vi "paramget.vi"(8 "dwLen":u32, 10 "byPara":u8) -> (1 "data out":u8[](array[numeric]), 2 "return":i32)   [LabVIEW 2016]
panel:
  in  "cmd_std_header_t":T1
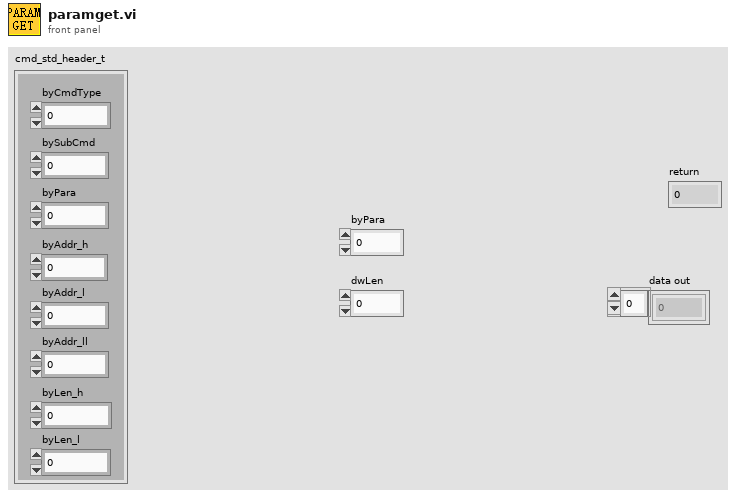
[diagram p1: front panel]
types:
  T1 = cluster{"byCmdType":u8, "bySubCmd":u8, "byPara":u8, "byAddr_h":u8, "byAddr_l":u8, "byAddr_ll":u8, "byLen_h":u8, "byLen_l":u8}
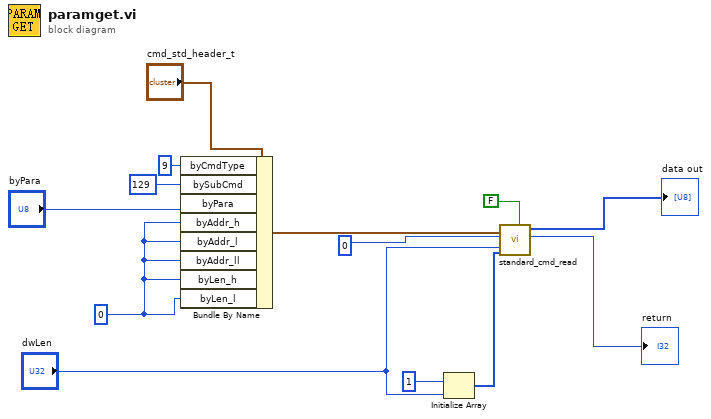
[diagram p0: block diagram]
diagram:
  w4 = u8 0
  n1 = Bundle By Name(cluster="cmd_std_header_t", "byCmdType"=u8 9, "bySubCmd"=u8 129, "byPara"="byPara", "byAddr_h"=w4, "byAddr_l"=w4, "byAddr_ll"=w4, "byLen_h"=w4, "byLen_l"=w4) -> (w12:T1)
  n2 = Initialize Array(u8 1, "dwLen") -> (w8:u8[])
  n3 = call "standard_cmd_read.vi"("COM"=FALSE, "data"=w8, "dwLen"="dwLen", "dwAddr"=u32 0, "cmd_std_header_t"=w12) -> ("return"=→"return":i32, "data out"=→"data out":u8[])  [unwired: 5 in]
